vi "Packet Sniffer Example.vi"() -> ()   [LabVIEW 2018]
doc: "This example project provides a library of VIs that work together to wrap various ethernet packet sniffing functions available from WinPcap, a Windows packet capture program.\n\nNote: You must install WinPcap before running this example. You can download WinPcap from www.winpcap.org.\n\nThis VI reads ethernet packets. It outputs the raw data for the packet as a hexadecimal string. It also parses out the ethernet and IP header information, as well as timestamp information for each packet.\n\nThis VI also enumerates all the ethernet adapters on your system and allows you interactively to select between the various adapters.\n\nPlease note that this project is for demonstration purposes only. It was designed to demonstrate one method in which LabVIEW can be used to interface with external software utilities (such as WinPcap). NI Engineers can only address questions on how to call external code from LabVIEW, not the contents of each call demonstrated in this example. In addition, we cannot guarantee that the software will work with newer versions of the external software package."
uses:
  control_packet_header_ethernet.ctl
  control_packet_header_ip.ctl
  lvwpcap.lvlib
panel:
  out "帧类型":string caption="以太网帧类型"
  out "时间标识":timestamp
  out "IP Header":T1 {"options / padding" format="%02x"; "fragment offset" format="%04x"; "IHL" format="%02x"; "version" format="%01x"; "type of service" format="%02x"; "total length" format="%02x"; "identification" format="%04x"; "flags" format="%.0x"; "time to live" format="%02x"; "protocol" format="%02.0f"; "header checksum" format="%04x"; "source address" format="%08x"; "destination address" format="%08x"}
  out "ethernet header":T2 {"destination MAC address"."?" format="%02x"; "destination MAC address"."?" format="%02x"; "destination MAC address"."?" format="%02x"; "destination MAC address"."?" format="%02x"; "destination MAC address"."?" format="%02x"; "destination MAC address"."?" format="%02x"; "source MAC address"."?" format="%02x"; "source MAC address"."?" format="%02x"; "source MAC address"."?" format="%02x"; "source MAC address"."?" format="%02x"; "source MAC address"."?" format="%02x"; "source MAC address"."?" format="%02x"; "length / type" format="%04x"}
  in  "Adapters":i32(listbox)
  out "ip data":string
  out "destination address":string
  out "source address":string
  out "IP Packet":bool
  out "timestamp":cluster{"tv_sec":u32, "tv_usec":u32}
  out "raw data":string
  out "packets":i32
  in  "stop":bool
  # "Timestamp"
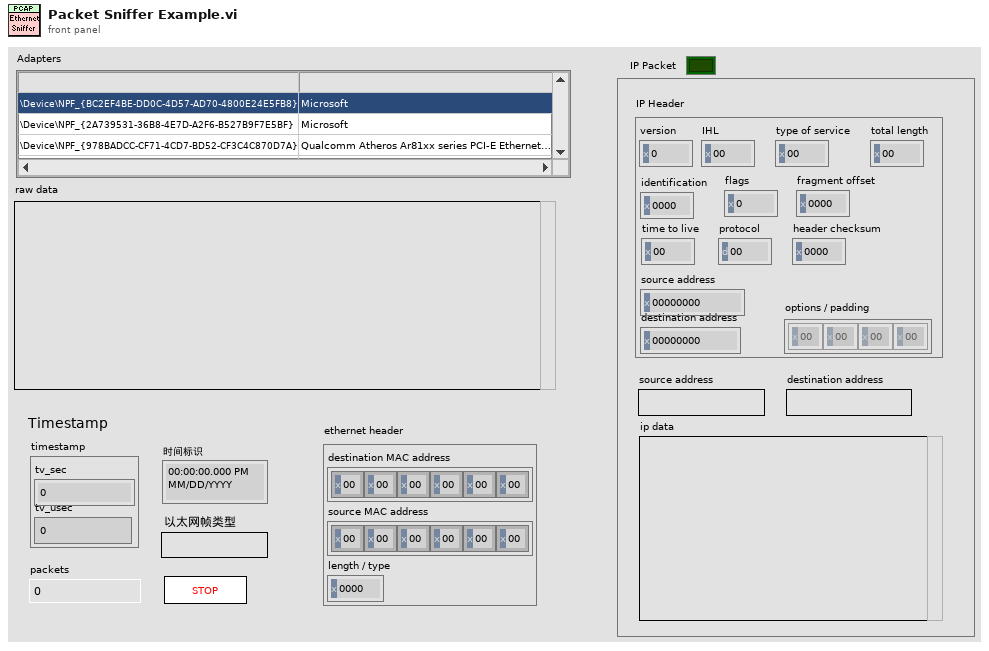
[diagram p1: front panel]
types:
  T1 = typedef "control_packet_header_ip.ctl" = cluster{"version":u8, "IHL":u8, "type of service":u8, "total length":u16, "identification":u16, "flags":u16, "fragment offset":u16, "time to live":u8, "protocol":u8, "header checksum":u16, "source address":u32, "destination address":u32, "options / padding":u8[]}
  T2 = typedef "control_packet_header_ethernet.ctl" = cluster{"destination MAC address":cluster{u8, u8, u8, u8, u8, u8}, "source MAC address":cluster{u8, u8, u8, u8, u8, u8}, "length / type":u16}
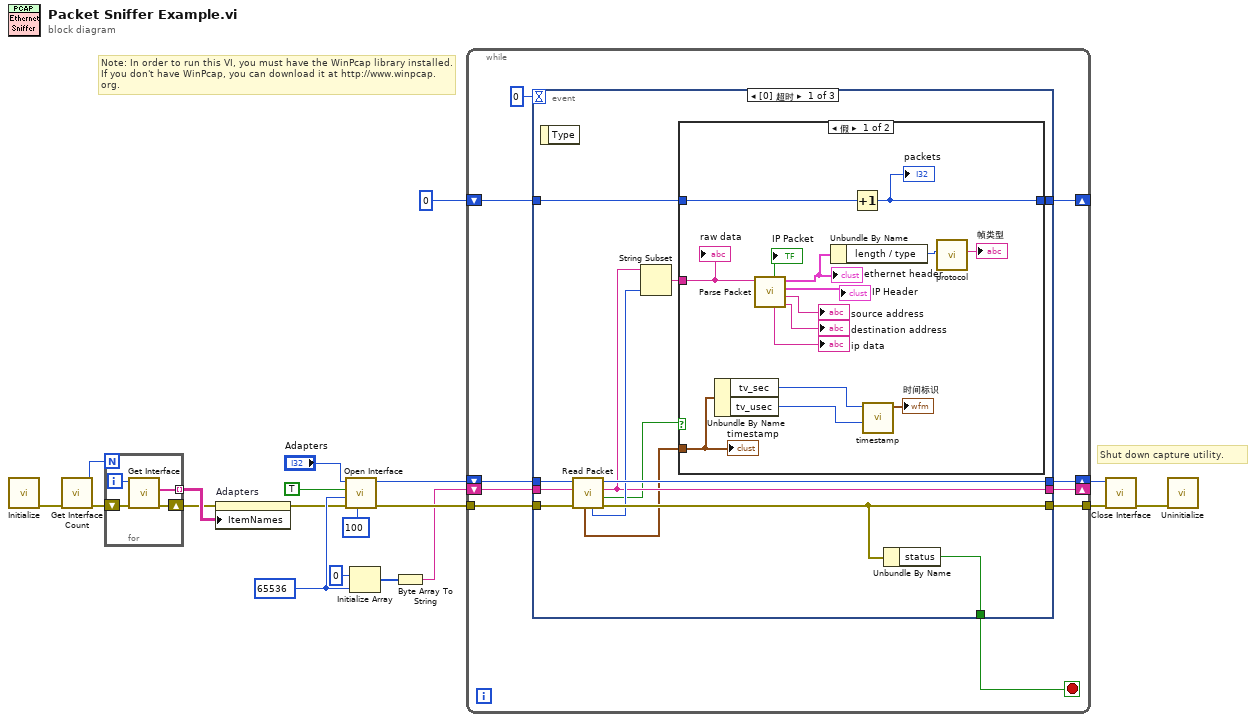
[diagram p0: block diagram]
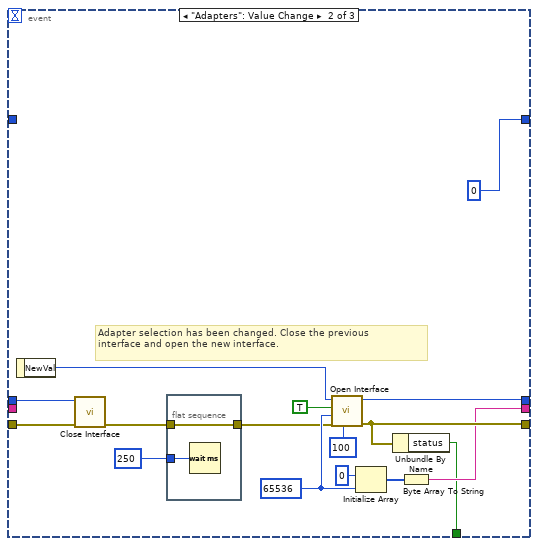
[diagram p3: hidden frame]
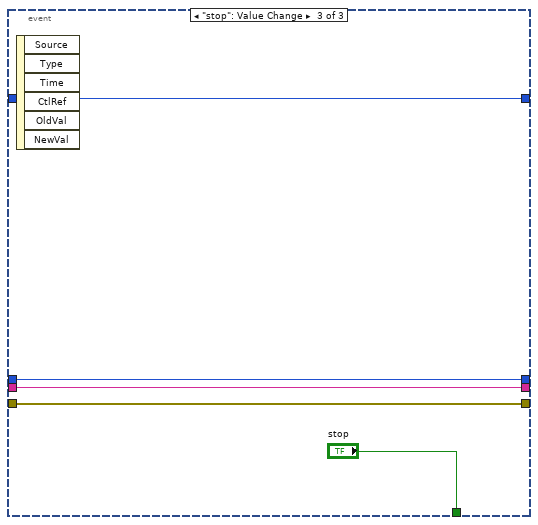
[diagram p4: hidden frame]
diagram:
  w14 = 65536 ("capture_size (65536)")
  # "Shut down capture utility."
  # "Note: In order to run this VI, you must have the WinPcap library installed. If you don't have WinPcap, you can download it at http://www.winpcap.org."
  n1 = call "Initialize.vi"() -> ("error out"=w8:errorcluster)  [unwired: 11 in]
  n2 = call "Get Interface Count.vi"("error in (no error)"=w8) -> ("error out"=w7:errorcluster, "count"=w6:i32)  [unwired: 9 in]
  n3 = for {
    N: w6 -> [_]
    shift-right: [w22] -> w2
    shift-left: w7 -> [w23]
    tunnel: [w20] -> w4 mode=indexing
    i -> [w21]
    n4 = call "Get Interface.vi"("error in (no error)"=w23, "index"=w21) -> ("error out"=w22:errorcluster, "lvwpcap_interface_array"=w20:string[])  [unwired: 8 in]
  }
  n5 = property on="Adapters" class="MCListbox (严格)"(error in=w2, "ItemNames"=w4) -> (error out=w1:errorcluster)  [unwired: 1 in, 1 out]
  n6 = call "Open Interface.vi"("read_timeout (1000)"=100, "error in (no error)"=w1, "capture_size (65536)"=w14, "promiscuous mode (T)"=TRUE, "adapter (0)"="Adapters") -> ("error out"=w18:errorcluster, "pcap reference"=w19:u32)  [unwired: 5 in]
  n7 = Initialize Array(u8 0, w14) -> (w12:u8[])
  n8 = Byte Array To String(unsigned byte array=w12) -> (string=w11:string)
  n9 = while {
    tunnel: w18 -> [w32]
    tunnel: [w31] -> w17
    shift-right: [w30] -> w16
    shift-left: w19 -> [w33]
    shift-right: [w28] -> _
    shift-left: w11 -> [w29]
    shift-right: [w26] -> _
    shift-left: 0 -> [w27]
    stop <- w25 stop-if-true
    n10 = event shown="[0] 超时" {
      selector: _ -> [_ _ _]
      dyn-events: _ -> [_ _ _]
      timeout: 0 -> [_ _ _]
      tunnel: w33 -> [w46 w65 w84]
      tunnel: w32 -> [w45 w77 w82]
      tunnel: [w44 w78 w82] -> w31
      tunnel: [w43 w75 w84] -> w30
      tunnel: w29 -> [w42 _ w83]
      tunnel: [w40 w70 w83] -> w28
      tunnel: w27 -> [w37 _ w81]
      tunnel: [w36 0 w81] -> w26
      tunnel: [w35 w68 "stop"] -> w25
      event Timeout {
        n11 = event-data() -> ()  [unwired: 1 in, 1 out]
        n12 = call "Read Packet.vi"("error in (no error)"=w45, "capture_data"=w42, "pcap reference"=w46) -> ("error out"=w44:errorcluster, "timed out"=w38:bool, "capture_data out"=w40:string, "pcap reference out"=w43:u32, "capture_len"=w41:u32, "timestamp"=w34:cluster{"tv_sec":u32, "tv_usec":u32})  [unwired: 3 in]
        n13 = String Subset(string=w40, length (rest)=w41) -> (substring=w39:string)  [unwired: 1 in]
        n14 = case shown="假" w38 {
          tunnel: w39 -> [w61 _]
          tunnel: w34 -> [w53 _]
          tunnel: w37 -> [w56 w62]
          tunnel: [w55 w62] -> w36
          frame False {
            n15 = Unbundle By Name(w53) -> ("tv_sec"=w48:u32, "tv_usec"=w47:u32)
            n16 = call "Parse Packet.vi"("data"=w61) -> ("destination address"=→"destination address":string, "source address"=→"source address":string, "ip header"=→"IP Header":T1, "ethernet header"=w51:T2, "ip data"=→"ip data":string, "ip packet"=→"IP Packet":bool)  [unwired: 5 in]
            "ethernet header" <- w51
            n17 = Unbundle By Name(w51) -> ("length / type"=w50:u16)
            n18 = Increment(x=w56) -> (x+1=w55:i32)
            "packets" <- w55
            n19 = call "timestamp.vi"("timestamp"=w48, "秒数的小数部分"=w47) -> ("时间标识"=→"时间标识":timestamp)  [unwired: 8 in]
            n20 = call "protocol.vi"("数值"=w50) -> ("字符串"=→"帧类型":string)  [unwired: 10 in]
            "raw data" <- w61
            "timestamp" <- w53
          }
          frame True {
            # "timed out"
          }
        }
        n21 = Unbundle By Name(w44) -> ("status"=w35:bool)
      }
      event "Adapters": Value Change {
        w71 = 65536 ("capture_size (65536)")
        # "Adapter selection has been changed. Close the previous\ninterface and open the new interface."
        n22 = event-data() -> ("NewVal"=w76:i32)  [unwired: 1 in]
        n23 = call "Close Interface.vi"("error in (no error)"=w77, "pcap reference"=w65) -> ("error out"=w64:errorcluster)  [unwired: 9 in]
        n24 = flat-sequence {
          tunnel: w64 -> [w80]
          tunnel: [w80] -> w63
          tunnel: u32 250 ("milliseconds to wait") -> [w79]
          frame #0 {
            n25 = Wait (ms)(milliseconds to wait=w79) -> ()  [unwired: 1 out]
          }
        }
        n26 = call "Open Interface.vi"("read_timeout (1000)"=100, "error in (no error)"=w63, "capture_size (65536)"=w71, "promiscuous mode (T)"=TRUE, "adapter (0)"=w76) -> ("error out"=w78:errorcluster, "pcap reference"=w75:u32)  [unwired: 5 in]
        n27 = Initialize Array(u8 0, w71) -> (w73:u8[])
        n28 = Unbundle By Name(w78) -> ("status"=w68:bool)
        n29 = Byte Array To String(unsigned byte array=w73) -> (string=w70:string)
      }
      event "stop": Value Change {
        n30 = event-data() -> ()  [unwired: 1 in, 6 out]
      }
    }
  }
  n31 = call "Close Interface.vi"("error in (no error)"=w17, "pcap reference"=w16) -> ("error out"=w15:errorcluster)  [unwired: 9 in]
  n32 = call "Uninitialize.vi"("error in (no error)"=w15) -> ()  [unwired: 10 in, 1 out]
